vi "Main - On Load - Mutation Code.vi"(8 "error in (no error)":errorcluster, 11 "Device Item Ref in":T1 format="%.0x") -> (0 "error out":errorcluster, 3 "Device Item Ref out":T1 format="%.0x")   [LabVIEW 2015, in "Waveform Data Logger System Explorer.lvlib"]
uses:
  Waveform Data Logger System Explorer.lvlib
  <vilib>/NI Veristand/Custom Device API/Custom Device Item Ref.ctl
  NationalInstruments.VeriStand.SystemDefinitionAPI
  Shared/Globals/Property Strings.vi
  Shared/Globals/Default Values.vi
  <vilib>/NI Veristand/Custom Device API/Set Item Property (Boolean).vi
  <vilib>/NI Veristand/Custom Device API/Set Item Property (I32).vi
  Shared/Globals/Global GUIDs.vi
  <vilib>/NI Veristand/Custom Device Tools/Custom Device Utility Library/NI VeriStand - Search for All Items by GUID.vi
  <vilib>/NI VeriStand/Custom Device API/Custom Device API.lvlib
  Shared/Waveform Data Logger Shared.lvlib
  <vilib>/NI VeriStand/Custom Device Tools/Custom Device Utility Library/Custom Device Utility Library.lvlib
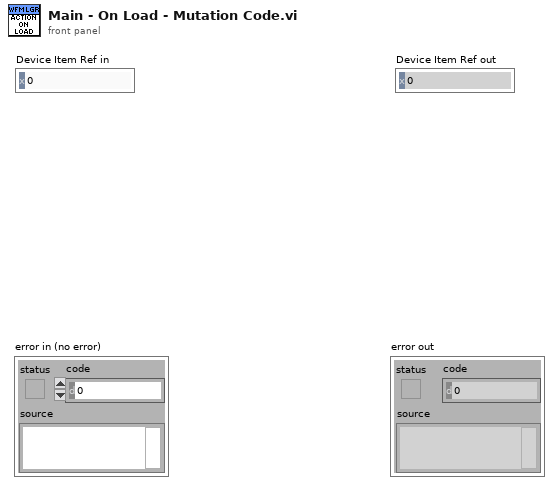
[diagram p1: front panel]
types:
  T1 = typedef "Custom Device API.lvlib/Custom Device Item Ref.ctl" = u64
  T2 = typedef "Custom Device API.lvlib/Custom Device Item Info.ctl" = cluster{"Name":string, "Is Channel":bool, "GUID":string, "Is Waveform":bool}
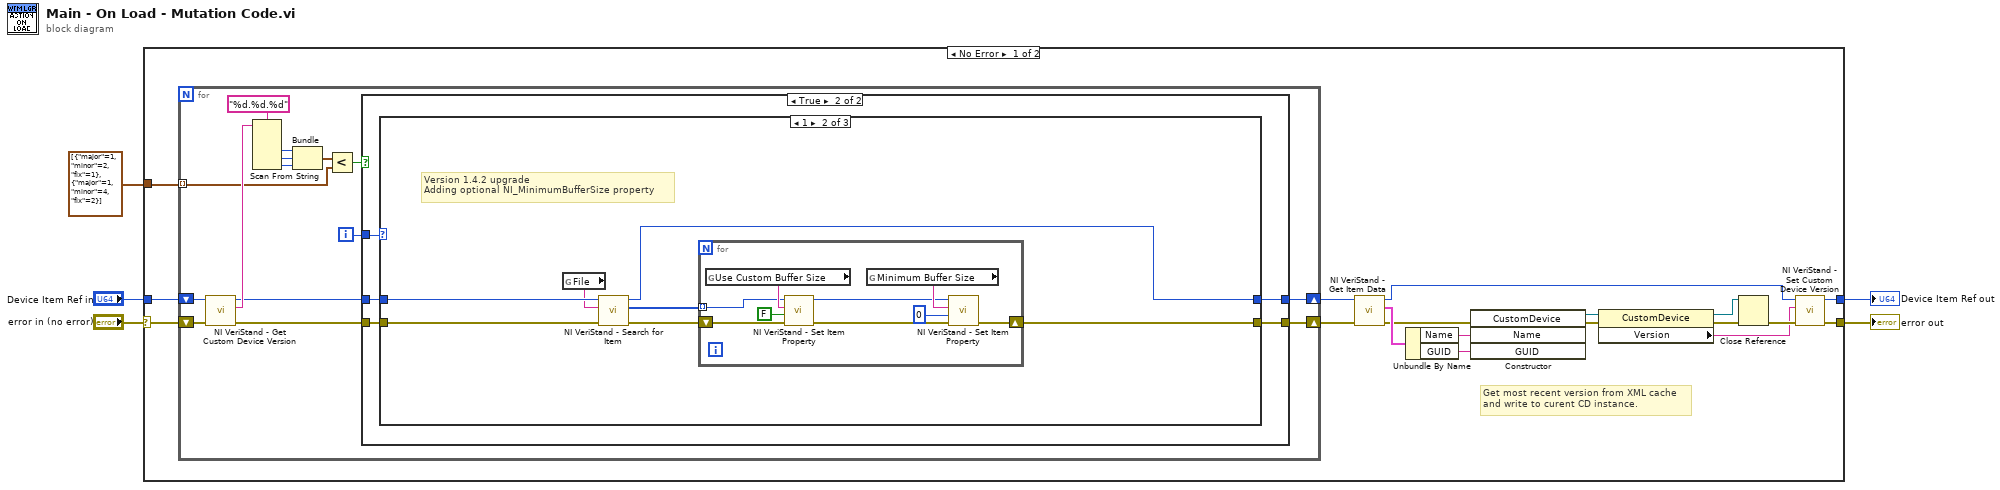
[diagram p0: block diagram]
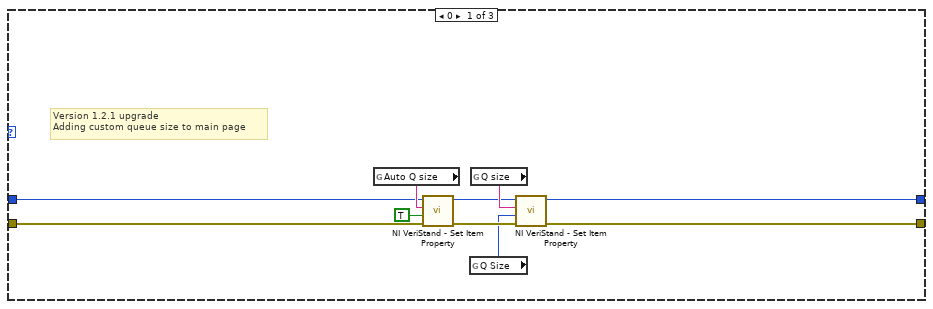
[diagram p3: hidden frame]
diagram:
  n1 = case shown="No Error" "error in (no error)" {
    selector: "error in (no error)" -> [w22 w75]
    tunnel: [w6 w75] -> w2
    tunnel: "Device Item Ref in" -> [w21 w74]
    tunnel: [w7 w74] -> w1
    tunnel: cluster{"major":i32, "minor":i32, "fix":i32}[] [{"major"=1, "minor"=2, "fix"=1}, {"major"=1, "minor"=4, "fix"=2}] -> [w23 _]
    frame No Error {
      # "Get most recent version from XML cache\nand write to curent CD instance."
      n2 = for {
        tunnel: w23 -> [w25] mode=indexing
        shift-right: [w29] -> w19
        shift-left: w22 -> [w34]
        shift-right: [w27] -> w20
        shift-left: w21 -> [w33]
        i -> [w26]
        n3 = call <vilib>:"NI VeriStand - Get Custom Device Version.vi"("error in (no error)"=w34, "Device Ref in"=w33) -> ("error out"=w30:errorcluster, "Value"=w32:string, "Device Ref out"=w28:T1)  [unwired: 7 in]
        n4 = Scan From String(format string="%d.%d.%d", input string=w32) -> (output 1=w36:i32, output 2=w37:i32, output 3=w24:i32)  [unwired: 5 in, 3 out]
        n5 = Bundle(w36, w37, w24) -> (w38:cluster{i32, i32, i32})  [unwired: 1 in]
        n6 = Less?(x=w38, y=w25) -> (x < y?=w31:bool)
        n7 = case shown="True" w31 {
          tunnel: w30 -> [w40 w45]
          tunnel: [w40 w44] -> w29
          tunnel: w28 -> [w39 w41]
          tunnel: [w39 w42] -> w27
          tunnel: w26 -> [_ w43]
          frame False {
          }
          frame True {
            n8 = case shown="1" w43 {
              tunnel: w45 -> [w48 w60 w73]
              tunnel: [w46 w62 w73] -> w44
              tunnel: [w47 w58 w72] -> w42
              tunnel: w41 -> [w49 w61 w72]
              frame 0 {
                # "Version 1.2.1 upgrade\nAdding custom queue size to main page"
                n9 = global read "Property Strings.vi" "Auto Q size"() -> (w51:string)
                n10 = call-poly <vilib>:"NI VeriStand - Set Item Property.vi"("error in (no error)"=w48, "Value"=TRUE, "Property Name"=w51, "Item Ref in"=w49) -> ("error out"=w53:errorcluster, "Item Ref out"=w52:T1)  [unwired: 5 in, 1 out]
                n11 = global read "Default Values.vi" "Q Size"() -> (w50:i32)
                n12 = global read "Property Strings.vi" "Q size"() -> (w54:string)
                n13 = call-poly <vilib>:"NI VeriStand - Set Item Property.vi"("error in (no error)"=w53, "Value"=w50, "Property Name"=w54, "Item Ref in"=w52) -> ("error out"=w46:errorcluster, "Item Ref out"=w47:T1)  [unwired: 5 in, 1 out]
              }
              frame 1 {
                # "Version 1.4.2 upgrade\nAdding optional NI_MinimumBufferSize property"
                n14 = global read "Global GUIDs.vi" "File"() -> (w56:string)
                n15 = call-poly <vilib>:"NI VeriStand - Search for Item.vi"("error in"=w60, "Item GUID"=w56, "Section Ref in"=w61) -> ("error out"=w59:errorcluster, "Item Refs"=w57:T1[], "Section Ref out"=w58:T1)  [unwired: 5 in, 1 out]
                n16 = for {
                  shift-right: [w67] -> w62
                  shift-left: w59 -> [w66]
                  tunnel: w57 -> [w64] mode=indexing
                  n17 = global read "Property Strings.vi" "Use Custom Buffer Size"() -> (w65:string)
                  n18 = call-poly <vilib>:"NI VeriStand - Set Item Property.vi"("error in (no error)"=w66, "Value"=FALSE, "Property Name"=w65, "Item Ref in"=w64) -> ("error out"=w69:errorcluster, "Item Ref out"=w68:T1)  [unwired: 5 in, 1 out]
                  n19 = global read "Property Strings.vi" "Minimum Buffer Size"() -> (w70:string)
                  n20 = call-poly <vilib>:"NI VeriStand - Set Item Property.vi"("error in (no error)"=w69, "Value"=0, "Property Name"=w70, "Item Ref in"=w68) -> ("error out"=w67:errorcluster)  [unwired: 5 in, 2 out]
                }
              }
              frame Default {
              }
            }
          }
        }
      }
      n21 = call <vilib>:"NI VeriStand - Get Item Data.vi"("error in (no error)"=w19, "Item Ref in"=w20) -> ("error out"=w11:errorcluster, "Item Info"=w12:T2, "Item Ref out"=w9:T1)  [unwired: 7 out]
      n22 = Unbundle By Name(w12) -> ("Name"=w14:string, "GUID"=w13:string)
      n23 = constructor class="CustomDevice"(error in=w11, "Name"=w14, "GUID"=w13) -> (reference out=w17:refnum<k24>, error out=w18:errorcluster)  [unwired: 2 in, 3 out]
      n24 = property class="CustomDevice"(reference=w17, error in=w18) -> (reference out=w15:refnum<k24>, error out=w16:errorcluster, "Version"=w8:string)
      n25 = Close Reference(reference=w15, error in (no error)=w16) -> (error out=w10:errorcluster)
      n26 = call <vilib>:"NI VeriStand - Set Custom Device Version.vi"("error in (no error)"=w10, "Value"=w8, "Device Ref in"=w9) -> ("error out"=w6:errorcluster, "Device Ref out"=w7:T1)  [unwired: 7 in]
    }
    frame Error {
    }
  }
  "error out" <- w2
  "Device Item Ref out" <- w1
